vi "connect_password.vi"(8 "error in (no error)":errorcluster, 9 "Connection Name":string, 10 "Password":T2, 11 "Connection Info.":T1={"Remote"="", "Username"="", "Port (22)"=22}) -> (0 "error out":errorcluster, 2 "isSshConnected":bool, 3 "Return String":string)   [LabVIEW 2022 SP3, in "LabSSH.lvlib"]
doc: "<License>This software is distributed under the BSD 3-Clause License. For the full license please see license.txt or visit www.labvolution.com/license</License>"
uses:
  LabSSH.lvlib
  Password..cluster.ctl
  Connection Info..cluster.ctl
  FGV State..enum.ctl
  D:/project/tvtEye/guard_tvt/tools/LabSSH Library/References/LabSSH.dll
  References/LabSSH.dll
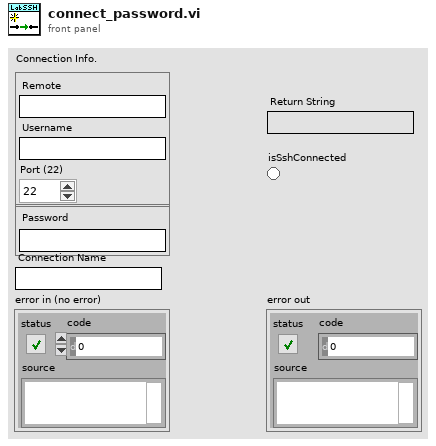
[diagram p1: front panel]
types:
  T1 = typedef "LabSSH.lvlib/Connection Info..cluster.ctl" = cluster{"Remote":string, "Username":string, "Port (22)":i32}
  T2 = typedef "LabSSH.lvlib/Password..cluster.ctl" = cluster{"Password":string}
  T3 = typedef "LabSSH.lvlib/FGV State..enum.ctl" = enum16{"GET", "SET"}
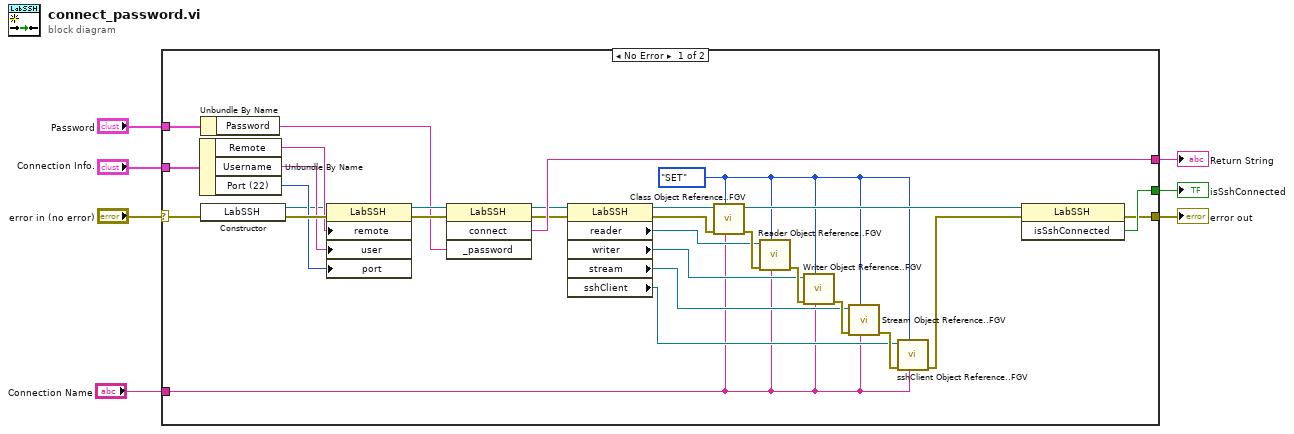
[diagram p0: block diagram]
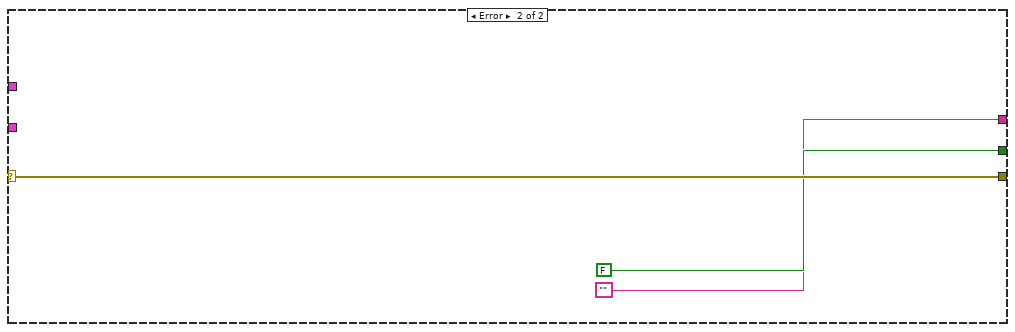
[diagram p2: hidden frame]
diagram:
  n1 = case shown="No Error" "error in (no error)" {
    selector: "error in (no error)" -> [w34 w40]
    tunnel: [w37 FALSE ("isSshConnected")] -> w7
    tunnel: "Password" -> [w36 _]
    tunnel: [w35 ""] -> w5
    tunnel: "Connection Info." -> [w29 _]
    tunnel: [w24 w40] -> w2
    tunnel: "Connection Name" -> [w9 _]
    frame No Error {
      w12 = FGV_State..enum."SET" ("FGV State")
      n2 = Unbundle By Name(w29) -> ("Remote"=w28:string, "Username"=w27:string, "Port (22)"=w26:i32)
      n3 = Unbundle By Name(w36) -> ("Password"=w10:string)
      n4 = constructor class="LabSSH" ("Constructor Node")(error in=w34) -> (reference out=w8:refnum<k24>, error out=w30:errorcluster)  [unwired: 2 in, 1 out]
      n5 = property on="Property Node" class="LabSSH"(reference=w8, error in=w30, "remote"=w28, "user"=w27, "port"=w26) -> (reference out=w33:refnum<k24>, error out=w31:errorcluster)
      n6 = invoke on="Invoke Node" class="LabSSH" method="connect"(reference=w33, error in=w31, "_password"=w10) -> (reference out=w25:refnum<k24>, error out=w32:errorcluster, "connect"=w35:string)  [unwired: 1 in, 1 out]
      n7 = property class="LabSSH"(reference=w25, error in=w32) -> (reference out=w23:refnum<k24>, error out=w21:errorcluster, "reader"=w16:refnum<k24>, "writer"=w15:refnum<k24>, "stream"=w14:refnum<k24>, "sshClient"=w13:refnum<k24>)
      n8 = call "Class Object Reference..FGV.vi"("Connection Name"=w9, "FGV State (GET)"=w12, "error in (no error)"=w21, "LabSSH ref in"=w23) -> ("error out"=w20:errorcluster, "LabSSH ref out"=w22:refnum<k24>)  [unwired: 6 in]
      n9 = call "Reader Object Reference..FGV.vi"("Connection Name"=w9, "FGV State (GET)"=w12, "error in (no error)"=w20, "Reader ref in"=w16) -> ("error out"=w19:errorcluster)  [unwired: 6 in, 1 out]
      n10 = call "Writer Object Reference..FGV.vi"("Connection Name"=w9, "FGV State (GET)"=w12, "error in (no error)"=w19, "Writer ref in"=w15) -> ("error out"=w18:errorcluster)  [unwired: 6 in, 1 out]
      n11 = call "Stream Object Reference..FGV.vi"("Connection Name"=w9, "FGV State (GET)"=w12, "error in (no error)"=w18, "Stream ref in"=w14) -> ("error out"=w17:errorcluster)  [unwired: 6 in, 1 out]
      n12 = call "sshClient Object Reference..FGV.vi"("Connection Name"=w9, "FGV State (GET)"=w12, "error in (no error)"=w17, "sshClient ref in"=w13) -> ("error out"=w11:errorcluster)  [unwired: 6 in, 1 out]
      n13 = invoke on="Invoke Node" class="LabSSH" method="isSshConnected"(reference=w22, error in=w11) -> (error out=w24:errorcluster, "isSshConnected"=w37:bool)  [unwired: 1 in, 1 out]
    }
    frame Error {
    }
  }
  "error out" <- w2
  "isSshConnected" <- w7
  "Return String" <- w5
